vi "Multistage Multirate Filter Continuous Processing.vi"() -> ()   [LabVIEW 2023]
doc: "Demonstrates how to use the DFD NStage MRate Filtering VI to process a signal continuously with a multistage multirate filter.\n\nComplete the following steps to use this VI.\n1) Select the <B>Filtering Mode</B>.\n2) Set the <B>Zero Phase?</B> value to True.\n3) Run the VI.\n4) Observe the Signal In and Signal Out plots to verify that no delay exists between them.\n5) Click the <B>STOP</B> button to stop this VI.\n6) Set the <B>Zero Phase?</B> value to False.\n7) Run the VI again.\n8) Observe the Signal In and Signal Out plots. Notice that a delay exists between them.\n9) Click the <B>STOP</B> button to stop this VI."
uses:
  <vilib>/addons/Digital Filter Design/_Objects.llb/DFD Multirate Filtering Mode.ctl
  <vilib>/addons/Digital Filter Design/Multirate.llb/DFD NStage MRate Filtering (Wfm).vi
  <vilib>/addons/Digital Filter Design/NI_DigFilterLicensed.lvlib
  <vilib>/measure/NI_MABase.lvlib
panel:
  out "Error Message":string
  in  "Filtering Mode":T1=2 items=["No Rate Change", "Interpolation", "Decimation"]
  out "Signals":waveform(dbl)[](graph)
  in  "Zero Phase?":bool=TRUE
  in  "stop":bool
  # "Select Help>>Show Context Help and move the cursor over the VI icon for more information."
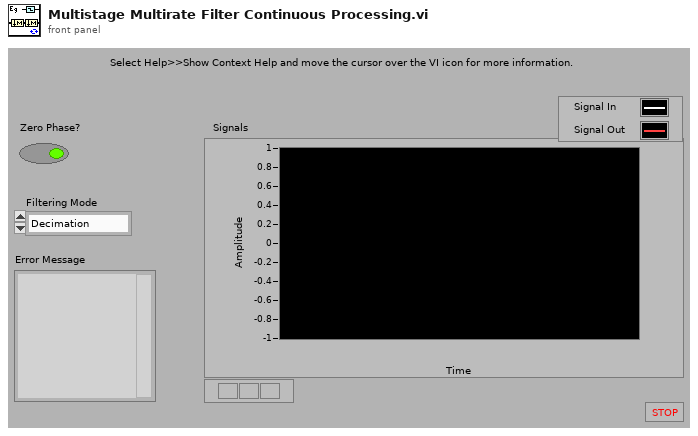
[diagram p1: front panel]
types:
  T1 = typedef "NI_DigFilterLicensed.lvlib/DFD Multirate Filtering Mode.ctl" = u16
  T2 = typedef "NI_DigFilterLicensed.lvlib/DFD Multirate Filter Obj.ctl" = cluster{"mMRate_Structure":enum16{"CIC", "FIR", "IIR", "Lattice"}, "mMRate_Mode":T3, "mMRate_Factor":i32, "mMRate_FIRParams":cluster{"mMRate_FIR_H":dbl[], "mMRate_FIR_IsNyquist?":bool, "mMRate_FIR_IsSymmetric?":bool}, "mMRate_CICParams":cluster{"mMRate_CIC_#Stage":i32, "mMRate_CIC_Lag":i32, "mMRate_CIC_Type":enum16{"Lowpass", "Highpass"}}, "mMRate_Order":i32, "mMRate_Version":string, "mMRate_Comments":string, "mMRate_RationalFactor":cluster{"mMRate_L":i32, "mMRate_M":i32}, "mMRate_Fs":dbl, "mMRate_Quantized?":bool, "mMRate_QFilterGain":dbl, "mMRate_CoefWl":i16, "mMRate_Scaling":cluster{"mMRate_ScaleByPowerOf2?":bool, "mMRate_ScaleType":T4}, "mMRate_InputWl":i16, "mMRate_OutputWl":i16, "mMRate_OutputMode":T5, "mMRate_MultMode":T6, "mMRate_BitPruning":bool, "mMRate_GainWl":i16, "mMRate_OutputFwl":i16, "mMRate_SumIwl":i16, "mMRate_InputIwl ":i16, "mMRate_SumWl":i16, "mMRate_CoefIwl":i16}
  T3 = typedef "NI_DigFilterLicensed.lvlib/DFD Multirate Mode.ctl" = i16
  T4 = typedef "NI_DigFilterLicensed.lvlib/DFD Coef Norm Type.ctl" = enum16{"No Norm", "Time Domain 1-Norm", "Time Domain 2-Norm", "Time Domain Inf-Norm"}
  T5 = typedef "NI_DigFilterLicensed.lvlib/DFD Round-off Mode.ctl" = enum16{"Nearest", "Truncation"}
  T6 = typedef "NI_DigFilterLicensed.lvlib/DFD FXP MRate Multiply Mode.ctl" = enum16{"Truncated", "Full"}
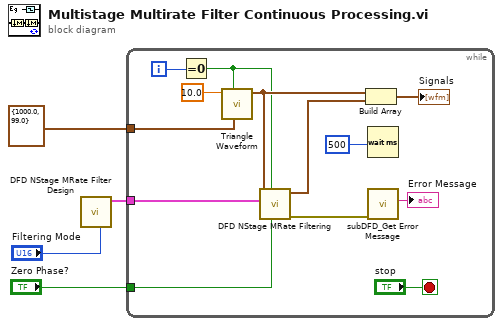
[diagram p0: block diagram]
diagram:
  n1 = call <vilib>:"DFD NStage MRate Filter Design.vi"("filtering mode"="Filtering Mode") -> ("multirate filters out"=w4:T2[])  [unwired: 7 in, 3 out]
  n2 = while {
    tunnel: w4 -> [w15]
    tunnel: "Zero Phase?" -> [w9]
    tunnel: cluster{"Fs":dbl, "#s":dbl} {"Fs"=1000.0, "#s"=99.0} ("sampling info") -> [w8]
    i -> [w14]
    stop <- "stop" stop-if-true
    n3 = Equal To 0?(x=w14) -> (x = 0?=w7:bool)
    n4 = call <vilib>:"Triangle Waveform.vi"("sampling info"=w8, "reset signal"=w7, "frequency"=10.0) -> ("signal out"=w13:waveform(dbl))  [unwired: 4 in, 4 out]
    n5 = call-poly <vilib>:"DFD NStage MRate Filtering.vi"("zero phase? (T)"=w9, "init? (F)"=w7, "multirate filters"=w15, "signal in"=w13) -> ("error out"=w6:errorcluster, "signal out"=w12:waveform(dbl))  [unwired: 1 in, 5 out]
    n6 = Build Array(w13, w12) -> (→"Signals":waveform(dbl)[])
    n7 = Wait (ms)(milliseconds to wait=u32 500 ("millisecond timer value")) -> ()  [unwired: 1 out]
    n8 = call <vilib>:"subDFD_Get Error Message.vi"("error in (no error)"=w6) -> ("Error Message"=→"Error Message":string)  [unwired: 10 out]
  }
